vi "CH4_Tx.vi"() -> ()   [LabVIEW 2018]
uses:
  Stream/Stream.lvclass
  RxTx/RxTx.lvclass
panel:
  in  "RxTx.lvclass":refnum<class "RxTx.lvclass">
  in  "Stream.lvclass":refnum<class "Stream.lvclass">
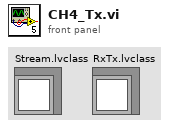
[diagram p1: front panel]
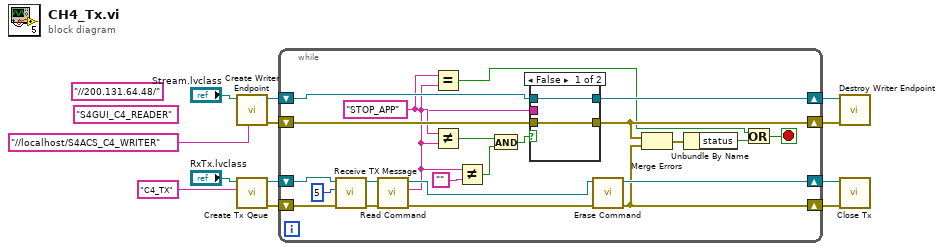
[diagram p0: block diagram]
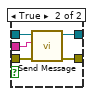
[diagram p2: hidden frame]
diagram:
  (unwired) "//200.131.64.48/" ("Reader Name")
  (unwired) "S4GUI_C4_READER" ("reader name")
  n1 = call "Create Writer Endpoint.vi"("writer name"="//localhost/S4ACS_C4_WRITER" ("reader name"), "Stream in"="Stream.lvclass") -> ("error out"=w3:errorcluster, "Stream out"=w5:refnum<class "Stream.lvclass">)  [unwired: 8 in]
  n2 = call "Create Tx Qeue.vi"("Writer Name"="C4_TX" ("Reader Name"), "RxTx in"="RxTx.lvclass") -> ("error out"=w10:errorcluster, "RxTx out"=w11:refnum<class "RxTx.lvclass">)  [unwired: 8 in]
  n3 = while {
    shift-right: [w26] -> w1
    shift-left: w3 -> [w28]
    shift-right: [w27] -> w12
    shift-left: w5 -> [w29]
    shift-right: [w21] -> w6
    shift-left: w10 -> [w30]
    shift-right: [w23] -> w7
    shift-left: w11 -> [w31]
    stop <- w18 stop-if-true
    w17 = "STOP_APP"
    n4 = call "Receive TX Message.vi"("error in (no error)"=w30, "timeout in ms"=5, "RxTx in"=w31) -> ("error out"=w34:errorcluster, "RxTx out"=w33:refnum<class "RxTx.lvclass">)  [unwired: 7 in]
    n5 = call "Read Command.vi"("error in (no error)"=w34, "RxTx in"=w33) -> ("error out"=w22:errorcluster, "Message"=w16:string, "RxTx out"=w24:refnum<class "RxTx.lvclass">)  [unwired: 7 in]
    n6 = Equal?(x=w17, y=w16) -> (x = y?=w20:bool)
    n7 = Not Equal?(x=w17, y=w16) -> (x != y?=w15:bool)
    n8 = Not Equal?(x=w16, y="") -> (x != y?=w14:bool)
    n9 = And(x=w15, y=w14) -> (x .and. y?=w13:bool)
    n10 = case shown="False" w13 {
      tunnel: w29 -> [w37 w42]
      tunnel: w28 -> [w36 w41]
      tunnel: [w37 w40] -> w27
      tunnel: w16 -> [_ w39]
      tunnel: [w36 w38] -> w26
      frame False {
      }
      frame True {
        n11 = call "Send Message.vi"("error in (no error)"=w41, "Message"=w39, "Stream in"=w42) -> ("error out"=w38:errorcluster, "Stream out"=w40:refnum<class "Stream.lvclass">)  [unwired: 7 in]
      }
    }
    n12 = call "Erase Command.vi"("error in (no error)"=w22, "RxTx in"=w24) -> ("error out"=w21:errorcluster, "RxTx out"=w23:refnum<class "RxTx.lvclass">)  [unwired: 8 in]
    n13 = Merge Errors(w26, w21) -> (w35:errorcluster)
    n14 = Unbundle By Name(w35) -> ("status"=w19:bool)
    n15 = Or(x=w20, y=w19) -> (x .or. y?=w18:bool)
  }
  n16 = call "Destroy Writer Endpoint.vi"("error in (no error)"=w1, "Stream in"=w12) -> ()  [unwired: 8 in, 2 out]
  n17 = call "Close Tx.vi"("error in (no error)"=w6, "RxTx in"=w7) -> ()  [unwired: 8 in, 2 out]
